vi "Unregister Logger.vi"(8 "error in (no error)":errorcluster, 10 "Unregister Logger":T1, 11 "Log Manager Module in":refnum<class "Log Manager Module.lvclass">) -> (0 "error out":errorcluster, 3 "Log Manager Module out":refnum<class "Log Manager Module.lvclass">)   [LabVIEW 2020, in "VolatusData.lvlib" / "Log Manager Module.lvclass"]
uses:
  Log Manager Module.lvclass
  Log Manager Module.lvclass/Log Manager Module.ctl
  Volatus/Module/Module.lvclass
  Volatus/Event Level.ctl
  Volatus/Volatus.lvlib
  Volatus/MessageQ/MessageQ.lvclass
  C:/dev/lv20CE/gpack-tests/lv-volatus/Volatus/Module/Module.lvclass
  C:/dev/lv20CE/gpack-tests/lv-volatus/VolatusData/Log Manager Module/Log Manager Module.lvclass
  Unregister Logger.ctl
  VolatusData.lvlib
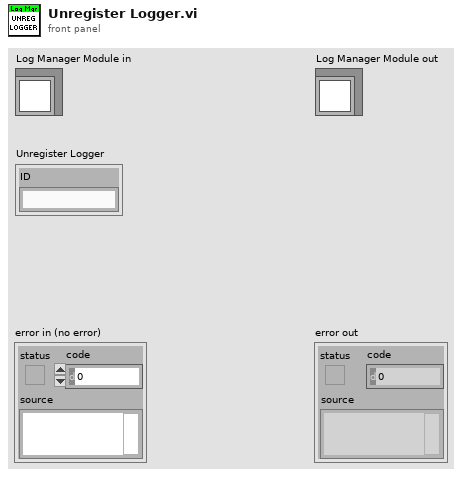
[diagram p1: front panel]
types:
  T1 = typedef "VolatusData.lvlib/Unregister Logger.ctl" = cluster{"ID":string}
  T2 = typedef "VolatusData.lvlib/Log Manager Module.lvclass/Group Info.ctl" = cluster{"Name":string, "Loggers":map{string, T3}}
  T3 = typedef "VolatusData.lvlib/Log Manager Module.lvclass/Logger.ctl" = cluster{"ID":string, "MsgQ":refnum<class "MessageQ.lvclass">, "State":T4, "Group":string}
  T4 = typedef "VolatusData.lvlib/Logger State.ctl" = enum16{"Unknown", "Idle", "Preparing", "Ready", "Logging", "Stopping"}
  T5 = typedef "Volatus.lvlib/Event Level.ctl" = enum16{"Debug", "Info", "Warning", "Error"}
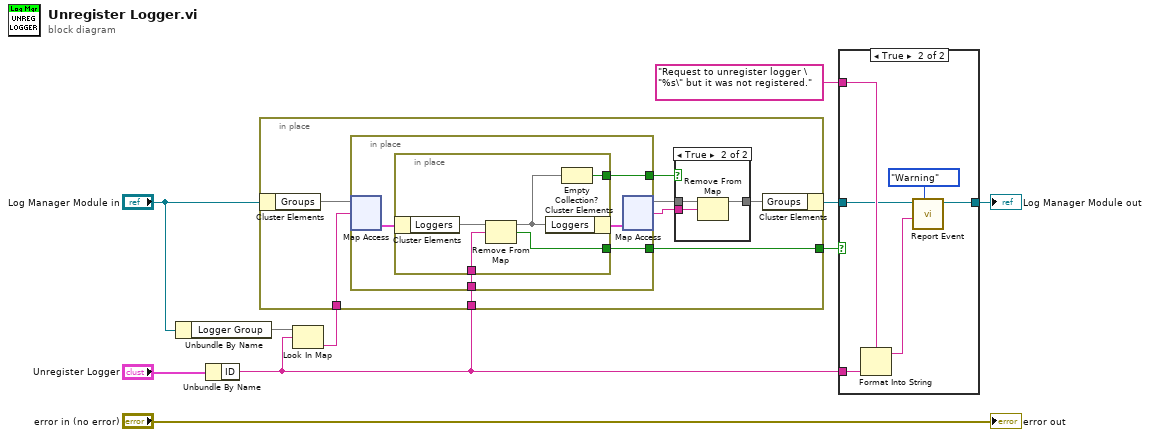
[diagram p0: block diagram]
diagram:
  n1 = Unbundle By Name("Log Manager Module in") -> ("Logger Group"=w3:map{string, string})
  n2 = Unbundle By Name("Unregister Logger") -> ("ID"=w2:string)
  n3 = Look In Map(map=w3, key=w2) -> (value=w1:string)  [unwired: 1 in, 1 out]
  n4 = in-place {
    in-place-border: w2 -> [w17]
    in-place-border: [w16] -> w8
    in-place-border: w1 -> [w11]
    n5 = in-place-cluster #1("Log Manager Module in") -> ("Groups"=w18:map{string, T2})
    n6 = in-place {
      in-place-border: w17 -> [w26]
      in-place-border: [w25] -> w16
      in-place-border: [w23] -> w12
      n7 = in-place-map #2(w18, w11) -> (w27:T2)  [unwired: 1 in, 1 out]
      n8 = in-place {
        in-place-border: w26 -> [w31]
        in-place-border: [w30] -> w25
        in-place-border: [w28] -> w23
        n9 = in-place-cluster #3(w27) -> ("Loggers"=w32:map{string, T3})
        n10 = Remove From Map(10:w31, 11:w32) -> (2:w30:bool, 3:w29:map{string, T3})  [unwired: 1 out]
        n11 = in-place-cluster #3("Loggers"=w29) -> (w24:T2)
        n12 = Empty Collection?(1:w29) -> (0:w28:bool)
      }
      n13 = in-place-map #2(w24) -> (w15:map{string, T2}, w14:string)  [unwired: 1 in, 1 out]
    }
    n14 = case shown="True" w12 {
      tunnel: w15 -> [w19 w22]
      tunnel: w14 -> [_ w21]
      tunnel: [w19 w20] -> w13
      frame False {
      }
      frame True {
        n15 = Remove From Map(10:w21, 11:w22) -> (3:w20:map{string, T2})  [unwired: 2 out]
      }
    }
    n16 = in-place-cluster #1("Groups"=w13) -> (w7:refnum<class "Log Manager Module.lvclass">)
  }
  n17 = case shown="True" w8 {
    tunnel: w2 -> [_ w39]
    tunnel: w7 -> [w33 w37]
    tunnel: "Request to unregister logger \"%s\" but it was not registered." -> [_ w38]
    tunnel: [w33 w35] -> w5
    frame False {
    }
    frame True {
      n18 = Format Into String(format string=w38, w39) -> (resulting string=w34:string)  [unwired: 2 in, 1 out]
      n19 = call "Report Event.vi"("Level (Info)"=Event_Level."Warning", "Message"=w34, "Module in"=w37) -> ("Module out"=w35:refnum<class "Log Manager Module.lvclass">)  [unwired: 7 in, 1 out]
    }
  }
  "Log Manager Module out" <- w5
  "error out" <- "error in (no error)"
